vi "Part 1.vi"(11 "Input":string) -> (3 "Output":i64)   [LabVIEW 2021]
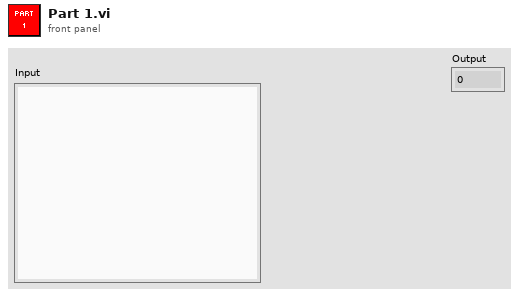
[diagram p1: front panel]
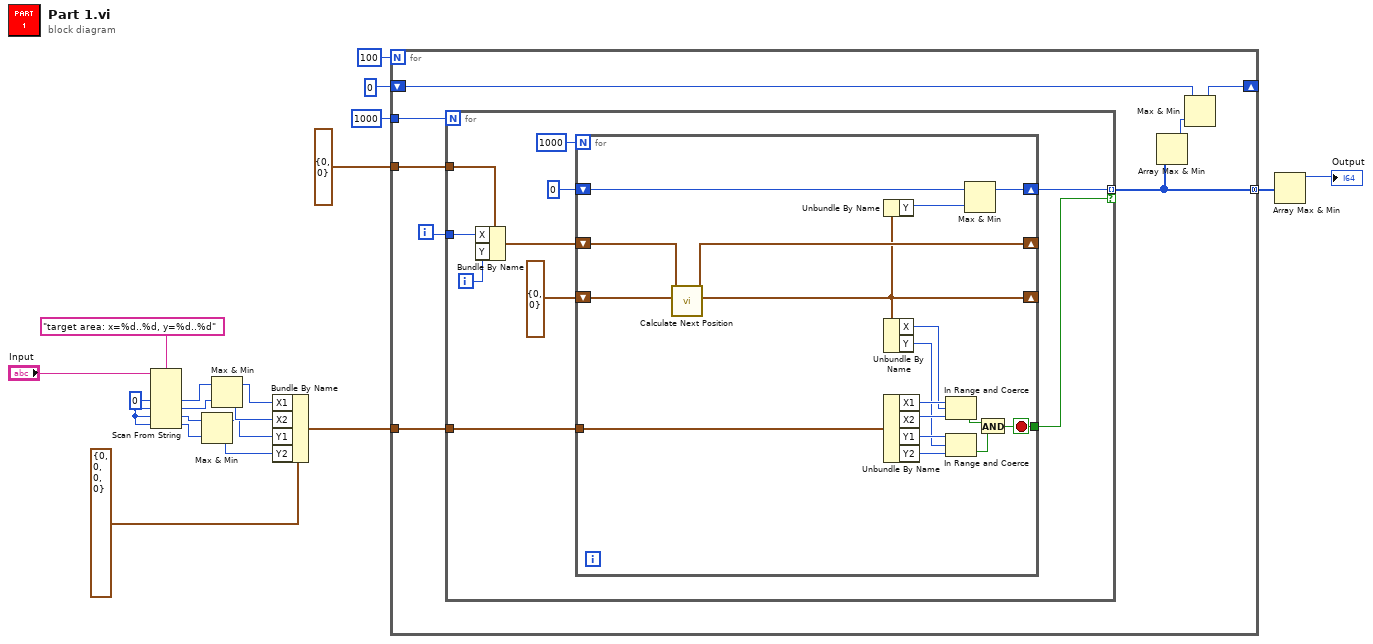
[diagram p0: block diagram]
diagram:
  w4 = i64 0 ("default value 1")
  n1 = Scan From String(format string="target area: x=%d..%d, y=%d..%d", input string="Input", default 1=w4, default 2=w4, default 3=w4, default 4=w4) -> (output 1=w14:i64, output 2=w12:i64, output 3=w10:i64, output 4=w8:i64)  [unwired: 2 in, 3 out]
  n2 = Max & Min(x=w10, y=w8) -> (max(x,y)=w9:i64, min(x,y)=w7:i64)
  n3 = Max & Min(x=w14, y=w12) -> (max(x,y)=w13:i64, min(x,y)=w11:i64)
  n4 = Bundle By Name(cluster=cluster{"X1":i64, "X2":i64, "Y1":i64, "Y2":i64} {"X1"=0, "X2"=0, "Y1"=0, "Y2"=0}, "X1"=w13, "X2"=w11, "Y1"=w9, "Y2"=w7) -> (w15:cluster{"X1":i64, "X2":i64, "Y1":i64, "Y2":i64})
  n5 = for {
    N: 100 -> [_]
    tunnel: 1000 -> [w27]
    tunnel: w15 -> [w26]
    tunnel: cluster{"X":i64, "Y":i64} {"X"=0, "Y"=0} -> [w25]
    tunnel: [w23] -> w6 mode=concatenating
    shift-right: [w20] -> _
    shift-left: i64 0 -> [w21]
    i -> [w24]
    n6 = for {
      N: w27 -> [_]
      tunnel: w26 -> [w37]
      tunnel: w25 -> [w36]
      tunnel: w24 -> [w34]
      tunnel: [w30] -> w23 mode=indexing if=w29
      i -> [w35]
      n7 = Bundle By Name(cluster=w36, "X"=w34, "Y"=w35) -> (w33:cluster{"X":i64, "Y":i64})
      n8 = for {
        N: 1000 -> [_]
        tunnel: w37 -> [w54]
        shift-right: [w38] -> _
        shift-left: cluster{"X":i64, "Y":i64} {"X"=0, "Y"=0} -> [w41]
        shift-right: [w39] -> _
        shift-left: w33 -> [w40]
        shift-right: [w43] -> w30
        shift-left: i64 0 -> [w44]
        tunnel: [w42] -> w29
        stop <- w42 stop-if-true
        n9 = call "Calculate Next Position.vi"("Position In"=w41, "Velocity In"=w40) -> ("Position Out"=w38:cluster{"X":i64, "Y":i64}, "Velocity Out"=w39:cluster{"X":i64, "Y":i64})  [unwired: 8 in]
        n10 = Unbundle By Name(w38) -> ("Y"=w45:i64)
        n11 = Unbundle By Name(w38) -> ("X"=w51:i64, "Y"=w48:i64)
        n12 = Unbundle By Name(w54) -> ("X1"=w53:i64, "X2"=w52:i64, "Y1"=w50:i64, "Y2"=w49:i64)
        n13 = In Range and Coerce(upper limit=w53, x=w51, lower limit=w52) -> (In Range?=w47:bool)  [unwired: 1 out]
        n14 = In Range and Coerce(upper limit=w50, x=w48, lower limit=w49) -> (In Range?=w46:bool)  [unwired: 1 out]
        n15 = Max & Min(x=w44, y=w45) -> (max(x,y)=w43:i64)  [unwired: 1 out]
        n16 = And(x=w47, y=w46) -> (x .and. y?=w42:bool)
      }
    }
    n17 = Array Max & Min(array=w23) -> (max value=w22:i64)  [unwired: 3 out]
    n18 = Max & Min(x=w21, y=w22) -> (max(x,y)=w20:i64)  [unwired: 1 out]
  }
  n19 = Array Max & Min(array=w6) -> (max value=→"Output":i64)  [unwired: 3 out]
